vi "comb_alu.vi"(2 "Control":T1, 3 "B":T4, 4 "A":T4) -> (0 "Flags":T3, 1 "Result":T2)   [LabVIEW 2013]
panel:
  # "0 if logical\n1 if arythmetical"
  # "R1"
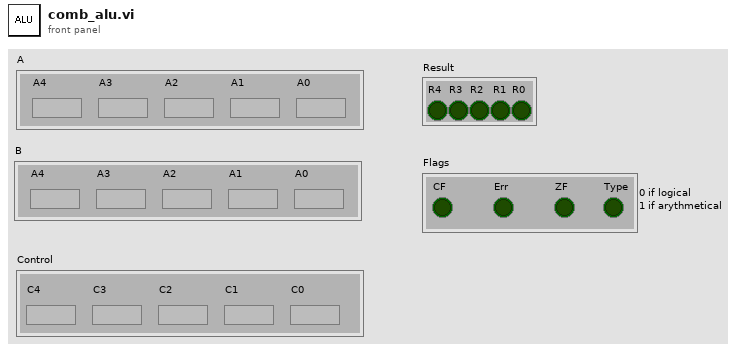
[diagram p1: front panel]
types:
  T1 = cluster{"C4":bool, "C3":bool, "C2":bool, "C1":bool, "C0":bool}
  T2 = cluster{"R4":bool, "R3":bool, "R2":bool, bool, "R0":bool}
  T3 = cluster{"CF":bool, "Err":bool, "ZF":bool, "Type":bool}
  T4 = cluster{"A4":bool, "A3":bool, "A2":bool, "A1":bool, "A0":bool}
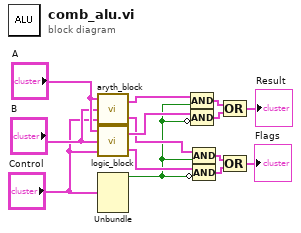
[diagram p0: block diagram]
diagram:
  n1 = call "aryth_block.vi"("Control"="Control", "B"="B", "A"="A") -> ("Flags"=w9:T3, "Result"=w1:T2)
  n2 = call "logic_block.vi"("Control"="Control", "B"="B", "A"="A") -> ("Flags"=w8:T3, "Result"=w10:T2)
  n3 = Unbundle("Control") -> ("C4"=w7:bool)  [unwired: 4 out]
  n4 = Compound Arithmetic op=AND(w1, w7) -> (w14:T2)
  n5 = Compound Arithmetic op=AND(w10, invert w7) -> (w11:T2)
  n6 = Compound Arithmetic op=AND(w9, w7) -> (w13:T3)
  n7 = Compound Arithmetic op=AND(w8, invert w7) -> (w12:T3)
  n8 = Compound Arithmetic op=OR(w14, w11) -> (→"Result":T2)
  n9 = Compound Arithmetic op=OR(w13, w12) -> (→"Flags":T3)
